vi "LSMcontroller_v66_improvedwfhandling.vi"() -> ()   [LabVIEW 2015] (continued)
                                tunnel: w3418 -> [_ w3423]
                                frame False {
                                }
                                frame True {
                                n926 = Quotient & Remainder(x=w3423, y=u32 2 ("min phot")) -> (floor(x/y)=w3422:u32)  [unwired: 1 out]
                                n927 = Max & Min(x=w3422, y=u32 5) -> (max(x,y)=w3421:u32)  [unwired: 1 out]
                                n928 = local write "min phot"(w3421) -> ()
                                }
                                }
                                n929 = To Double Precision Float(number=w3408) -> (double precision float=w3409:dbl)
                                n930 = local write "img_CH1"(w3410) -> ()
                                n931 = property on="img_CH1" class="IntGraph (strict)"("ZScale.Maximum"=w3409) -> ()  [unwired: 2 in, 2 out]
                                }
                                }
                                }
                                frame #4 {
                                w3427 = u16 1 items=["Stream to disk", "Post process", "real time process"] ("Ring")
                                n932 = local read "T3R Data processing"() -> (w3426:u16)
                                n933 = Equal?(x=w3426, y=w3427) -> (x = y?=w3425:bool)
                                n934 = case shown="False" w3425 {
                                frame False {
                                # "intensity"
                                n935 = local read "Current Average"() -> (w3432:sgl)
                                n936 = local read "image2list"() -> (w3428:u16)
                                n937 = local read "image1list"() -> (w3429:u16)
                                n938 = call "dattoimage.vi"("image2list"=w3428, "Current Average"=w3432, "image1list"=w3429) -> ("image 1 array out"=w3431:sgl[][])  [unwired: 1 out]
                                n939 = Transpose 2D Array(2D array=w3431) -> (transposed array=w3430:sgl[][])
                                n940 = local write "img_CH2"(w3430) -> ()
                                }
                                frame True {
                                }
                                }
                                }
                                }
                              }
                              frame Enabled {
                              }
                            }
                          }
                        }
                        n941 = local write "64bit disabled"(TRUE ("64bit disabled")) -> ()
                      }
                      frame #9 {
                        n942 = call "2pparameters.vi"("command"="get") -> ("params out"=w3435:T10)  [unwired: 1 in]
                        n943 = Unbundle By Name(w3435) -> ("auto OD"=w3434:bool)
                        n944 = case shown="True" w3434 {
                          frame False {
                          }
                          frame True {
                            n945 = call "configuration.vi"("command"="get") -> ("config out"=w3438:T11)  [unwired: 2 in, 1 out]
                            n946 = call "2pparameters.vi"("command"="get") -> ("params out"=w3441:T10)  [unwired: 1 in]
                            n947 = Unbundle By Name(w3438) -> ("image OD"=w3436:u16)
                            n948 = Unbundle By Name(w3441) -> ("ODfilt"=w3437:u16)
                            n949 = call "filterwheelcontrol_nothorlabslib.vi"("Current OD filt"=w3436, "New ODfilt"=w3437) -> ()  [unwired: 1 in]
                          }
                        }
                        n950 = call "reset AO_DO_v3.vi"() -> ()  [unwired: 12 in]
                      }
                      frame #10 {
                        n951 = stacked-sequence {
                          tunnel: w3455 -> [w3458 _ _ _ _ _]
                          tunnel: w3454 -> [w3457 _ _ _ _ _]
                          tunnel: w3453 -> [w3456 _ _ _ _ _]
                          tunnel: w3452 -> [_ w3507 _ _ _ _]
                          tunnel: w3451 -> [_ w3506 w3561 w3658 _ _]
                          tunnel: w3450 -> [_ w3505 w3560 w3657 _ _]
                          tunnel: w3449 -> [_ _ w3559 _ _ _]
                          tunnel: w3448 -> [_ _ w3558 _ _ _]
                          tunnel: w3447 -> [_ _ _ w3656 _ _]
                          tunnel: w3446 -> [_ _ _ w3655 _ _]
                          tunnel: w3445 -> [_ _ w3556 _ _ _]
                          tunnel: w3444 -> [_ _ w3555 _ _ _]
                          tunnel: w3443 -> [_ _ _ w3653 _ _]
                          tunnel: w3442 -> [_ _ _ w3652 _ _]
                          frame #0 {
                            n952 = case shown="False" w3458 {
                              tunnel: w3457 -> [_ w3480]
                              tunnel: w3456 -> [_ w3479]
                              frame True {
                                n953 = stacked-sequence {
                                seq-local: [w3459 _ _] -> [_ w3471 w3476]
                                frame #0 {
                                n954 = call "configuration.vi"("command"="get") -> ("config out"=w3465:T11)  [unwired: 2 in, 1 out]
                                n955 = Unbundle By Name(w3465) -> ("Voltage to Xgalvo"=w3462:i32)
                                n956 = call "2pparameters.vi"("command"="get") -> ("params out"=w3463:T10)  [unwired: 1 in]
                                n957 = in-place {
                                in-place-border: w3462 -> [w3470]
                                in-place-border: [w3467] -> w3459
                                n958 = in-place-cluster #9(w3463) -> ("aAO"=w3469:u32[])
                                n959 = call "remove channel from active arrayv2.vi"("line array in"=w3469, "line to remove"=w3470) -> ("line array out"=w3468:u32[], "index"=w3467:i32)  [unwired: 1 out]
                                n960 = in-place-cluster #9("aAO"=w3468) -> (w3460:T10)
                                }
                                n961 = call "2pparameters.vi"("Params in"=w3460, "command"="set") -> ()  [unwired: 1 out]
                                }
                                frame #1 {
                                n962 = call "waveformparamsv2.vi"("command"="rem AO", "index"=w3471) -> ()  [unwired: 3 in, 3 out]
                                }
                                frame #2 {
                                n963 = call "waveformsAObuffer.vi"("command"="get") -> ("AO wf out"=w3477:waveform(dbl)[])  [unwired: 1 in]
                                n964 = Delete From Array(array=w3477, length=1, index=w3476) -> (array with subset deleted=w3473:waveform(dbl)[])  [unwired: 1 out]
                                n965 = call "waveformsAObuffer.vi"("AO wf in"=w3473, "command"="set") -> ()  [unwired: 1 out]
                                }
                                }
                              }
                              frame False {
                                n966 = stacked-sequence {
                                seq-local: [w3481 _ _] -> [_ w3489 w3500]
                                tunnel: w3480 -> [_ w3488 _]
                                tunnel: w3479 -> [_ _ w3499]
                                frame #0 {
                                n967 = call "configuration.vi"("command"="get") -> ("config out"=w3486:T11)  [unwired: 2 in, 1 out]
                                n968 = Unbundle By Name(w3486) -> ("Voltage to Xgalvo"=w3482:i32)
                                n969 = call "2pparameters.vi"("command"="get") -> ("params out"=w3485:T10)  [unwired: 1 in]
                                n970 = Unbundle By Name(w3485) -> ("aAO"=w3483:u32[])
                                n971 = Search 1D Array(1D array=w3483, element=w3482) -> (index of element=w3481:i32)  [unwired: 1 in]
                                }
                                frame #1 {
                                n972 = call "waveformparamsv2.vi"("command"="get") -> ("Params out"=w3492:T14)  [unwired: 4 in, 2 out]
                                n973 = in-place {
                                in-place-border: w3489 -> [w3496]
                                in-place-border: w3488 -> [w3495]
                                n974 = in-place-cluster #10(w3492) -> ("AO parameters"=w3497:T15)
                                n975 = in-place {
                                in-place-border: w3495 -> [w3498]
                                n976 = in-place-array #11(w3497, w3496) -> ()  [unwired: 1 out]
                                n977 = in-place-array #11(w3498) -> (w3494:T15)  [unwired: 1 out]
                                }
                                n978 = in-place-cluster #10("AO parameters"=w3494) -> (w3490:T14)
                                }
                                n979 = call "waveformparamsv2.vi"("command"="set", "Params in"=w3490) -> ()  [unwired: 3 in, 3 out]
                                }
                                frame #2 {
                                n980 = call "waveformsAObuffer.vi"("command"="get") -> ("AO wf out"=w3503:waveform(dbl)[])  [unwired: 1 in]
                                n981 = Replace Array Subset(array=w3503, new element=w3499, index=w3500) -> (w3501:waveform(dbl)[])
                                n982 = call "waveformsAObuffer.vi"("AO wf in"=w3501, "command"="set") -> ()  [unwired: 1 out]
                                }
                                }
                              }
                            }
                          }
                          frame #1 {
                            n983 = case shown="True" w3507 {
                              tunnel: w3506 -> [_ w3529]
                              tunnel: w3505 -> [_ w3528]
                              frame True {
                                n984 = stacked-sequence {
                                seq-local: [w3508 _ _] -> [_ w3520 w3525]
                                frame #0 {
                                n985 = call "configuration.vi"("command"="get") -> ("config out"=w3514:T11)  [unwired: 2 in, 1 out]
                                n986 = Unbundle By Name(w3514) -> ("Voltage to Ygalvo"=w3511:i32)
                                n987 = call "2pparameters.vi"("command"="get") -> ("params out"=w3512:T10)  [unwired: 1 in]
                                n988 = in-place {
                                in-place-border: w3511 -> [w3519]
                                in-place-border: [w3516] -> w3508
                                n989 = in-place-cluster #12(w3512) -> ("aAO"=w3518:u32[])
                                n990 = call "remove channel from active arrayv2.vi"("line array in"=w3518, "line to remove"=w3519) -> ("line array out"=w3517:u32[], "index"=w3516:i32)  [unwired: 1 out]
                                n991 = in-place-cluster #12("aAO"=w3517) -> (w3509:T10)
                                }
                                n992 = call "2pparameters.vi"("Params in"=w3509, "command"="set") -> ()  [unwired: 1 out]
                                }
                                frame #1 {
                                n993 = call "waveformparamsv2.vi"("command"="rem AO", "index"=w3520) -> ()  [unwired: 3 in, 3 out]
                                }
                                frame #2 {
                                n994 = call "waveformsAObuffer.vi"("command"="get") -> ("AO wf out"=w3526:waveform(dbl)[])  [unwired: 1 in]
                                n995 = Delete From Array(array=w3526, length=1, index=w3525) -> (array with subset deleted=w3522:waveform(dbl)[])  [unwired: 1 out]
                                n996 = call "waveformsAObuffer.vi"("AO wf in"=w3522, "command"="set") -> ()  [unwired: 1 out]
                                }
                                }
                              }
                              frame False {
                                n997 = stacked-sequence {
                                seq-local: [w3530 _ _] -> [_ w3538 w3549]
                                tunnel: w3529 -> [_ w3537 _]
                                tunnel: w3528 -> [_ _ w3548]
                                frame #0 {
                                n998 = call "configuration.vi"("command"="get") -> ("config out"=w3535:T11)  [unwired: 2 in, 1 out]
                                n999 = Unbundle By Name(w3535) -> ("Voltage to Ygalvo"=w3531:i32)
                                n1000 = call "2pparameters.vi"("command"="get") -> ("params out"=w3534:T10)  [unwired: 1 in]
                                n1001 = Unbundle By Name(w3534) -> ("aAO"=w3532:u32[])
                                n1002 = Search 1D Array(1D array=w3532, element=w3531) -> (index of element=w3530:i32)  [unwired: 1 in]
                                }
                                frame #1 {
                                n1003 = call "waveformparamsv2.vi"("command"="get") -> ("Params out"=w3541:T14)  [unwired: 4 in, 2 out]
                                n1004 = in-place {
                                in-place-border: w3538 -> [w3545]
                                in-place-border: w3537 -> [w3544]
                                n1005 = in-place-cluster #13(w3541) -> ("AO parameters"=w3546:T15)
                                n1006 = in-place {
                                in-place-border: w3544 -> [w3547]
                                n1007 = in-place-array #14(w3546, w3545) -> ()  [unwired: 1 out]
                                n1008 = in-place-array #14(w3547) -> (w3543:T15)  [unwired: 1 out]
                                }
                                n1009 = in-place-cluster #13("AO parameters"=w3543) -> (w3539:T14)
                                }
                                n1010 = call "waveformparamsv2.vi"("command"="set", "Params in"=w3539) -> ()  [unwired: 3 in, 3 out]
                                }
                                frame #2 {
                                n1011 = call "waveformsAObuffer.vi"("command"="get") -> ("AO wf out"=w3552:waveform(dbl)[])  [unwired: 1 in]
                                n1012 = Replace Array Subset(array=w3552, new element=w3548, index=w3549) -> (w3550:waveform(dbl)[])
                                n1013 = call "waveformsAObuffer.vi"("AO wf in"=w3550, "command"="set") -> ()  [unwired: 1 out]
                                }
                                }
                              }
                            }
                          }
                          frame #2 {
                            n1014 = Build Array(w3556, w3555) -> (w3554:bool[])
                            n1015 = Boolean Array To Number(Boolean array=w3554) -> (number=w3557:u32)
                            n1016 = case shown="0" w3557 {
                              tunnel: w3561 -> [_ _ w3604]
                              tunnel: w3560 -> [_ _ w3603]
                              tunnel: w3559 -> [_ w3583 w3601]
                              tunnel: w3558 -> [_ w3582 w3602]
                              frame 1, Default {
                                n1017 = stacked-sequence {
                                seq-local: [w3562 _ _] -> [_ w3574 w3579]
                                frame #0 {
                                n1018 = call "configuration.vi"("command"="get") -> ("config out"=w3568:T11)  [unwired: 2 in, 1 out]
                                n1019 = Unbundle By Name(w3568) -> ("2P shutter"=w3565:i32)
                                n1020 = call "2pparameters.vi"("command"="get") -> ("params out"=w3566:T10)  [unwired: 1 in]
                                n1021 = in-place {
                                in-place-border: w3565 -> [w3573]
                                in-place-border: [w3570] -> w3562
                                n1022 = in-place-cluster #15(w3566) -> ("aDO"=w3572:u32[])
                                n1023 = call "remove channel from active arrayv2.vi"("line array in"=w3572, "line to remove"=w3573) -> ("line array out"=w3571:u32[], "index"=w3570:i32)  [unwired: 1 out]
                                n1024 = in-place-cluster #15("aDO"=w3571) -> (w3563:T10)
                                }
                                n1025 = call "2pparameters.vi"("Params in"=w3563, "command"="set") -> ()  [unwired: 1 out]
                                }
                                frame #1 {
                                n1026 = call "waveformparamsv2.vi"("command"="rem DO", "index"=w3574) -> ()  [unwired: 3 in, 3 out]
                                }
                                frame #2 {
                                n1027 = call "waveformsDObuffer.vi"("command"="get") -> ("DO wf out"=w3580:digitalwaveform[])  [unwired: 1 in]
                                n1028 = Delete From Array(array=w3580, length=1, index=w3579) -> (array with subset deleted=w3576:digitalwaveform[])  [unwired: 1 out]
                                n1029 = call "waveformsDObuffer.vi"("DO wf in"=w3576, "command"="set") -> ()  [unwired: 1 out]
                                }
                                }
                              }
                              frame 2 {
                                n1030 = stacked-sequence {
                                tunnel: w3583 -> [_ w3594 _]
                                tunnel: w3582 -> [_ _ w3598]
                                frame #0 {
                                n1031 = call "configuration.vi"("command"="get") -> ("config out"=w3585:T11)  [unwired: 2 in, 1 out]
                                n1032 = call "2pparameters.vi"("command"="get") -> ("params out"=w3589:T10)  [unwired: 1 in]
                                n1033 = Unbundle By Name(w3585) -> ("2P shutter"=w3584:i32)
                                n1034 = in-place {
                                in-place-border: w3584 -> [w3593]
                                n1035 = in-place-cluster #16(w3589) -> ("aDO"=w3592:u32[])
                                n1036 = call "add channel to active arrayv2.vi"("line array in"=w3592, "line to add"=w3593) -> ("line array out"=w3591:u32[])  [unwired: 2 out]
                                n1037 = in-place-cluster #16("aDO"=w3591) -> (w3587:T10)
                                }
                                n1038 = call "2pparameters.vi"("Params in"=w3587, "command"="set") -> ()  [unwired: 1 out]
                                }
                                frame #1 {
                                n1039 = call "waveformparamsv2.vi"("command"="add DO", "add DO"=w3594) -> ()  [unwired: 3 in, 3 out]
                                }
                                frame #2 {
                                n1040 = call "waveformsDObuffer.vi"("command"="get") -> ("DO wf out"=w3599:digitalwaveform[])  [unwired: 1 in]
                                n1041 = Build Array (concatenate)(w3599, w3598) -> (w3597:digitalwaveform[])
                                n1042 = call "waveformsDObuffer.vi"("DO wf in"=w3597, "command"="set") -> ()  [unwired: 1 out]
                                }
                                }
                              }
                              frame 0 {
                                n1043 = stacked-sequence {
                                seq-local: [w3605 _ _] -> [_ w3613 w3635]
                                tunnel: w3604 -> [_ _ _]
                                tunnel: w3603 -> [_ _ _]
                                tunnel: w3602 -> [_ _ w3634]
                                tunnel: w3601 -> [_ w3612 _]
                                frame #0 {
                                n1044 = call "configuration.vi"("command"="get") -> ("config out"=w3610:T11)  [unwired: 2 in, 1 out]
                                n1045 = call "2pparameters.vi"("command"="get") -> ("params out"=w3609:T10)  [unwired: 1 in]
                                n1046 = Unbundle By Name(w3610) -> ("2P shutter"=w3606:i32)
                                n1047 = Unbundle By Name(w3609) -> ("aDO"=w3607:u32[])
                                n1048 = Search 1D Array(1D array=w3607, element=w3606) -> (index of element=w3605:i32)  [unwired: 1 in]
                                }
                                frame #1 {
                                n1049 = call "2pparameters.vi"("command"="get") -> ("params out"=w3616:T10)  [unwired: 1 in]
                                n1050 = Unbundle By Name(w3616) -> ("wavdet"=w3614:bool, "autoshutter"=w3615:bool)
                                n1051 = case shown="True" w3615 {
                                tunnel: w3613 -> [_ w3620]
                                tunnel: w3614 -> [_ w3619]
                                tunnel: w3612 -> [_ w3618]
                                frame False {
                                }
                                frame True {
                                n1052 = case shown="False" w3619 {
                                tunnel: w3620 -> [w3624 _]
                                tunnel: w3618 -> [w3622 _]
                                frame False {
                                n1053 = Index Array(array=w3622, index=0) -> (element=w3621:T18)
                                n1054 = call "waveformparamsv2.vi"("command"="get") -> ("Params out"=w3627:T14)  [unwired: 4 in, 2 out]
                                n1055 = in-place {
                                in-place-border: w3624 -> [w3631]
                                in-place-border: w3621 -> [w3629]
                                n1056 = in-place-cluster #17(w3627) -> ("DO parameters"=w3632:T17)
                                n1057 = in-place {
                                in-place-border: w3629 -> [w3633]
                                n1058 = in-place-array #18(w3632, w3631) -> ()  [unwired: 1 out]
                                n1059 = in-place-array #18(w3633) -> (w3630:T17)  [unwired: 1 out]
                                }
                                n1060 = in-place-cluster #17("DO parameters"=w3630) -> (w3625:T14)
                                }
                                n1061 = call "waveformparamsv2.vi"("command"="set", "Params in"=w3625) -> ()  [unwired: 3 in, 3 out]
                                }
                                frame True {
                                }
                                }
                                }
                                }
                                }
                                frame #2 {
                                n1062 = call "2pparameters.vi"("command"="get") -> ("params out"=w3638:T10)  [unwired: 1 in]
                                n1063 = Unbundle By Name(w3638) -> ("wavdet"=w3636:bool, "autoshutter"=w3637:bool)
                                n1064 = case shown="True" w3637 {
                                tunnel: w3635 -> [_ w3642]
                                tunnel: w3636 -> [_ w3641]
                                tunnel: w3634 -> [_ w3640]
                                frame False {
                                }
                                frame True {
                                n1065 = case shown="False" w3641 {
                                tunnel: w3642 -> [w3646 _]
                                tunnel: w3640 -> [w3645 _]
                                frame False {
                                n1066 = Index Array(array=w3645, index=0) -> (element=w3643:digitalwaveform)
                                n1067 = call "waveformsDObuffer.vi"("command"="get") -> ("DO wf out"=w3648:digitalwaveform[])  [unwired: 1 in]
                                n1068 = Replace Array Subset(array=w3648, new element=w3643, index=w3646) -> (w3650:digitalwaveform[])
                                n1069 = call "waveformsDObuffer.vi"("DO wf in"=w3650, "command"="set") -> ()  [unwired: 1 out]
                                }
                                frame True {
                                }
                                }
                                }
                                }
                                }
                                }
                              }
                            }
                          }
                          frame #3 {
                            n1070 = Build Array(w3653, w3652) -> (w3654:bool[])
                            n1071 = Boolean Array To Number(Boolean array=w3654) -> (number=w3651:u32)
                            n1072 = case shown="0" w3651 {
                              tunnel: w3658 -> [_ _ w3701]
                              tunnel: w3657 -> [_ _ w3700]
                              tunnel: w3656 -> [_ w3680 w3698]
                              tunnel: w3655 -> [_ w3679 w3699]
                              frame 1, Default {
                                n1073 = stacked-sequence {
                                seq-local: [w3659 _ _] -> [_ w3671 w3676]
                                frame #0 {
                                n1074 = call "configuration.vi"("command"="get") -> ("config out"=w3665:T11)  [unwired: 2 in, 1 out]
                                n1075 = Unbundle By Name(w3665) -> ("LT timestamp"=w3662:u32)
                                n1076 = call "2pparameters.vi"("command"="get") -> ("params out"=w3663:T10)  [unwired: 1 in]
                                n1077 = in-place {
                                in-place-border: w3662 -> [w3670]
                                in-place-border: [w3667] -> w3659
                                n1078 = in-place-cluster #19(w3663) -> ("aDO"=w3669:u32[])
                                n1079 = call "remove channel from active arrayv2.vi"("line array in"=w3669, "line to remove"=w3670) -> ("line array out"=w3668:u32[], "index"=w3667:i32)  [unwired: 1 out]
                                n1080 = in-place-cluster #19("aDO"=w3668) -> (w3660:T10)
                                }
                                n1081 = call "2pparameters.vi"("Params in"=w3660, "command"="set") -> ()  [unwired: 1 out]
                                }
                                frame #1 {
                                n1082 = call "waveformparamsv2.vi"("command"="rem DO", "index"=w3671) -> ()  [unwired: 3 in, 3 out]
                                }
                                frame #2 {
                                n1083 = call "waveformsDObuffer.vi"("command"="get") -> ("DO wf out"=w3677:digitalwaveform[])  [unwired: 1 in]
                                n1084 = Delete From Array(array=w3677, length=1, index=w3676) -> (array with subset deleted=w3673:digitalwaveform[])  [unwired: 1 out]
                                n1085 = call "waveformsDObuffer.vi"("DO wf in"=w3673, "command"="set") -> ()  [unwired: 1 out]
                                }
                                }
                              }
                              frame 2 {
                                n1086 = stacked-sequence {
                                tunnel: w3680 -> [_ _ w3693]
                                tunnel: w3679 -> [_ w3691 _]
                                frame #0 {
                                n1087 = call "configuration.vi"("command"="get") -> ("config out"=w3682:T11)  [unwired: 2 in, 1 out]
                                n1088 = Unbundle By Name(w3682) -> ("LT timestamp"=w3681:u32)
                                n1089 = call "2pparameters.vi"("command"="get") -> ("params out"=w3686:T10)  [unwired: 1 in]
                                n1090 = in-place {
                                in-place-border: w3681 -> [w3690]
                                n1091 = in-place-cluster #20(w3686) -> ("aDO"=w3689:u32[])
                                n1092 = call "add channel to active arrayv2.vi"("line array in"=w3689, "line to add"=w3690) -> ("line array out"=w3688:u32[])  [unwired: 2 out]
                                n1093 = in-place-cluster #20("aDO"=w3688) -> (w3684:T10)
                                }
                                n1094 = call "2pparameters.vi"("Params in"=w3684, "command"="set") -> ()  [unwired: 1 out]
                                }
                                frame #1 {
                                n1095 = call "waveformparamsv2.vi"("command"="add DO", "add DO"=w3691) -> ()  [unwired: 3 in, 3 out]
                                }
                                frame #2 {
                                n1096 = call "waveformsDObuffer.vi"("command"="get") -> ("DO wf out"=w3696:digitalwaveform[])  [unwired: 1 in]
                                n1097 = Build Array (concatenate)(w3696, w3693) -> (w3695:digitalwaveform[])
                                n1098 = call "waveformsDObuffer.vi"("DO wf in"=w3695, "command"="set") -> ()  [unwired: 1 out]
                                }
                                }
                              }
                              frame 0 {
                                n1099 = stacked-sequence {
                                seq-local: [w3702 _ _] -> [_ w3712 w3729]
                                tunnel: w3701 -> [_ _ _]
                                tunnel: w3700 -> [_ _ _]
                                tunnel: w3699 -> [_ w3709 _]
                                tunnel: w3698 -> [_ _ w3728]
                                frame #0 {
                                n1100 = call "configuration.vi"("command"="get") -> ("config out"=w3707:T11)  [unwired: 2 in, 1 out]
                                n1101 = Unbundle By Name(w3707) -> ("LT timestamp"=w3703:u32)
                                n1102 = call "2pparameters.vi"("command"="get") -> ("params out"=w3706:T10)  [unwired: 1 in]
                                n1103 = Unbundle By Name(w3706) -> ("aDO"=w3704:u32[])
                                n1104 = Search 1D Array(1D array=w3704, element=w3703) -> (index of element=w3702:i32)  [unwired: 1 in]
                                }
                                frame #1 {
                                n1105 = local read "Measurement"() -> (w3711:T4)
                                n1106 = To Unsigned Long Integer(number=w3711) -> (unsigned 32bit integer=w3710:u32)
                                n1107 = case shown="5..7" w3710 {
                                tunnel: w3712 -> [_ w3716]
                                tunnel: w3709 -> [_ w3713]
                                frame 0..4, Default {
                                }
                                frame 5..7 {
                                n1108 = Index Array(array=w3713, index=0) -> (element=w3714:T18)
                                n1109 = call "waveformparamsv2.vi"("command"="get") -> ("Params out"=w3719:T14)  [unwired: 4 in, 2 out]
                                n1110 = in-place {
                                in-place-border: w3716 -> [w3723]
                                in-place-border: w3714 -> [w3721]
                                n1111 = in-place-cluster #21(w3719) -> ("DO parameters"=w3724:T17)
                                n1112 = in-place {
                                in-place-border: w3721 -> [w3725]
                                n1113 = in-place-array #22(w3724, w3723) -> ()  [unwired: 1 out]
                                n1114 = in-place-array #22(w3725) -> (w3722:T17)  [unwired: 1 out]
                                }
                                n1115 = in-place-cluster #21("DO parameters"=w3722) -> (w3717:T14)
                                }
                                n1116 = call "waveformparamsv2.vi"("command"="set", "Params in"=w3717) -> ()  [unwired: 3 in, 3 out]
                                }
                                }
                                }
                                frame #2 {
                                n1117 = local read "Measurement"() -> (w3727:T4)
                                n1118 = To Unsigned Long Integer(number=w3727) -> (unsigned 32bit integer=w3726:u32)
                                n1119 = case shown="5..7" w3726 {
                                tunnel: w3729 -> [_ w3733]
                                tunnel: w3728 -> [_ w3731]
                                frame 0..4, Default {
                                }
                                frame 5..7 {
                                n1120 = Index Array(array=w3731, index=0) -> (element=w3730:digitalwaveform)
                                n1121 = call "waveformsDObuffer.vi"("command"="get") -> ("DO wf out"=w3735:digitalwaveform[])  [unwired: 1 in]
                                n1122 = Replace Array Subset(array=w3735, new element=w3730, index=w3733) -> (w3737:digitalwaveform[])
                                n1123 = call "waveformsDObuffer.vi"("DO wf in"=w3737, "command"="set") -> ()  [unwired: 1 out]
                                }
                                }
                                }
                                }
                              }
                            }
                          }
                          frame #4 {
                            n1124 = call "Used AO lines.vi"() -> ("used AO names"=w3740:string[], "used AO lines"=w3738:tag[])  [unwired: 2 in]
                            n1125 = control-ref of="Analog Lines Plot"() -> (w3739:refnum<vi>)
                            n1126 = control-ref of="Digital Lines Plot"() -> (w3741:refnum<vi>)
                            n1127 = call "Used DO lines.vi"() -> ("used DO names"=w3742:string[], "used DO lines"=w3743:tag[])  [unwired: 2 in]
                            n1128 = local write "Analog Used Lines"(w3738) -> ()
                            n1129 = local write "Analog Used Names"(w3740) -> ()
                            n1130 = local write "Digital Used Lines"(w3743) -> ()
                            n1131 = local write "Digital Used Names"(w3742) -> ()
                            n1132 = call "prepDOWaveplot.vi"("DigitalGraph in"=w3741, "used DO names"=w3742) -> ()  [unwired: 1 in]
                            n1133 = call "prepAOWaveplot.vi"("WaveformGraph in"=w3739, "Analog Used Names"=w3740) -> ()  [unwired: 1 in]
                          }
                          frame #5 {
                            n1134 = local read "Meastab"() -> (w3758:enum32{"X-Y Image", "Linescan", "Timetrace"})
                            n1135 = property on="refwf" class="Ring (strict)"() -> ("RingText.Text"=w3755:string)  [unwired: 2 in, 2 out]
                            n1136 = case shown="\"Timetrace\"" w3758 {
                              tunnel: [w3760 w3761] -> w3759
                              frame "X-Y Image", Default {
                                n1137 = local read "Sampling rate"() -> (w3760:dbl)
                              }
                              frame "Timetrace" {
                                n1138 = local read "srateAODOtt"() -> (w3761:dbl)
                              }
                            }
                            n1139 = call "waveformsAObuffer.vi"("command"="get") -> ("AO wf out"=w3746:waveform(dbl)[])  [unwired: 1 in]
                            n1140 = local read "wavdet"() -> (w3756:bool)
                            n1141 = call "waveformsDObuffer.vi"("command"="get") -> ("DO wf out"=w3750:digitalwaveform[])  [unwired: 1 in]
                            n1142 = call "correctwaveformsizetemp.vi"("new sampling frequency (Hz)"=w3759, "start"=FALSE, "reference waveforms to"=w3755, "Analog waveforms in"=w3746, "stop"=TRUE, "Digital waveforms in"=w3750) -> ("analog wf out"=w3752:waveform(dbl)[], "Digital wf out"=w3754:digitalwaveform[], "measpoints"=w3757:i32)
                            n1143 = local write "Analog Lines Plot"(w3752) -> ()
                            n1144 = call "GetNumCamFramesv2.vi"("Digital Waveform Graph"=w3754) -> ("Numeric"=w3753:i32)  [unwired: 10 in]
                            n1145 = local write "Digital Lines Plot"(w3754) -> ()
                            n1146 = call "waveformsDObuffer.vi"("DO wf in"=w3754, "command"="set") -> ()  [unwired: 1 out]
                            n1147 = call "waveformsAObuffer.vi"("AO wf in"=w3752, "command"="set") -> ()  [unwired: 1 out]
                            n1148 = local write "Total Camera Frames"(w3753) -> ()
                            n1149 = case shown="True" w3756 {
                              tunnel: w3757 -> [_ w3762]
                              frame False {
                              }
                              frame True {
                                n1150 = local write "# of frames"(w3762) -> ()
                              }
                            }
                          }
                        }
                        n1151 = call "stoperaseCI.vi"() -> ()  [unwired: 12 in]
                        n1152 = call "stoperaseDO_img.vi"() -> ()  [unwired: 12 in]
                        n1153 = call "stoperaseAO_img.vi"() -> ()  [unwired: 12 in]
                        n1154 = call "stoperaseAI_img.vi"() -> ()  [unwired: 12 in]
                      }
                      frame #11 {
                        w3770 = FALSE ("Value (Signaling)")
                        n1155 = local read "save\ndata"() -> (w3763:bool)
                        n1156 = local read "save\ndata"() -> (w3764:bool)
                        n1157 = property on="Stop" class="Bool (strict)"("Visible"=FALSE, "DisabledEnum"=T7."Disabled" ("Disabled")) -> ()  [unwired: 2 in, 2 out]
                        n1158 = case shown="True" w3763 {
                          frame False {
                          }
                          frame True {
                            n1159 = call "closetiffs.vi"() -> ()  [unwired: 12 in]
                          }
                        }
                        n1160 = case shown="True" w3764 {
                          tunnel: w3765 -> [_ w3771]
                          frame False {
                          }
                          frame True {
                            n1161 = local read "filename prefix"() -> (w3773:string)
                            n1162 = local read "data dir"() -> (w3772:path)
                            n1163 = call "savetimestamps.vi"("timestamp"=w3771, "filename prefix in"=w3773, "data dir in"=w3772) -> ()  [unwired: 1 in]
                            n1164 = call "saveparams.vi"("filename prefix in"=w3773, "data dir in"=w3772) -> ()  [unwired: 2 in]
                          }
                        }
                        n1165 = property on="Start" class="Bool (strict)"("Visible"=TRUE, "DisabledEnum"=T7."Enabled" ("Disabled")) -> ()  [unwired: 2 in, 2 out]
                        n1166 = property on="Start" class="Bool (strict)"("Val(Sgnl)"=w3770) -> ()  [unwired: 2 in, 2 out]
                        n1167 = property on="Stop" class="Bool (strict)"("Val(Sgnl)"=w3770) -> ()  [unwired: 2 in, 2 out]
                      }
                      frame #12 {
                        w3777 = T21 2 items=["no dialog", "OK message", "continue or stop message", "OK message + warnings", "continue/stop + warnings"] ("type of dialog (OK msg:1)")
                        n1168 = call "displayerrors.vi"() -> ("error IO"=w3776:errorcluster)
                        n1169 = call <vilib>:"General Error Handler.vi"("type of dialog (OK msg:1)"=w3777, "error in (no error)"=w3776) -> ("error out"=w3775:errorcluster)  [unwired: 9 in, 4 out]
                        n1170 = call <vilib>:"Clear Errors.vi"("error in (no error)"=w3775) -> ("error out"=w3774:errorcluster)  [unwired: 5 in, 1 out]
                        n1171 = call "seterrors.vi"("error IO"=w3774) -> ()
                      }
                    }
                  }
                  frame "X-Y-Z-t movie" {
                    n1172 = call "2pparameters.vi"("command"="get") -> ("params out"=w3780:T10)  [unwired: 1 in]
                    n1173 = Bundle By Name(cluster=w3780, "type"="X-Y-Z-t movie") -> (w3778:T10)
                    n1174 = call "2pparameters.vi"("Params in"=w3778, "command"="set") -> ()  [unwired: 1 out]
                  }
                  frame "linescan" {
                    n1175 = call "2pparameters.vi"("command"="get") -> ("params out"=w3785:T10)  [unwired: 1 in]
                    n1176 = Bundle By Name(cluster=w3785, "type"="linescan") -> (w3787:T10)
                    n1177 = call "2pparameters.vi"("Params in"=w3787, "command"="set") -> ()  [unwired: 1 out]
                  }
                  frame "Timetrace", "Lifetime (contour)" {
                    n1178 = local read "ttt"() -> (w3788:T3)
                    n1179 = case shown="\"Point\", \"Resonant Ellipse\", \"freeform contour\", \"Fill Ellipse\", Default" w3788 {
                      selector: w3788 -> [_ w3789]
                      frame "Line" {
                      }
                      frame "Point", "Resonant Ellipse", "freeform contour", "Fill Ellipse", Default {
                        n1180 = stacked-sequence {
                          seq-local: [w3805 _ _ _ _ _ _ _ _ _ _] -> [_ _ w4678 _ _ w4691 w4758 _ _ w5118 _]
                          seq-local: [w3804 _ _ _ _ _ _ _ _ _ _] -> [_ _ _ _ _ _ _ _ w4805 _ _]
                          seq-local: [w3803 _ _ _ _ _ _ _ _ _ _] -> [_ _ _ _ _ _ _ _ w4804 _ _]
                          seq-local: [w3802 _ _ _ _ _ _ _ _ _ _] -> [_ _ _ _ _ _ _ _ w4807 _ _]
                          seq-local: [w3801 _ _ _ _ _ _ _ _ _ _] -> [_ _ _ _ _ _ _ _ w4803 _ _]
                          seq-local: [w3800 _ _ _ _ _ _ _ _ _ _] -> [_ _ _ _ _ _ _ _ w4802 _ _]
                          seq-local: [w3799 _ _ _ _ _ _ _ _ _ _] -> [_ _ _ _ _ _ _ _ w4806 _ _]
                          seq-local: [w3798 _ _ _ _ _ _ _ _ _ _] -> [_ _ _ _ _ _ _ _ w4801 _ _]
                          seq-local: [w3797 _ _ _ _ _ _ _ _ _ _] -> [_ _ _ _ _ _ _ _ w4800 _ _]
                          seq-local: [w3796 _ _ _ _ _ _ _ _ _ _] -> [_ _ _ _ _ _ _ _ w4795 _ _]
                          seq-local: [w3795 _ _ _ _ _ _ _ _ _ _] -> [_ _ _ _ _ _ _ _ w4794 _ _]
                          seq-local: [w3794 _ _ _ _ _ _ _ _ _ _] -> [_ _ _ _ _ _ _ _ w4799 _ _]
                          seq-local: [w3793 _ _ _ _ _ _ _ _ _ _] -> [_ _ _ _ _ _ _ _ w4798 _ _]
                          seq-local: [w3792 _ _ _ _ _ _ _ _ _ _] -> [_ _ _ _ _ _ _ _ w4797 _ _]
                          seq-local: [w3791 _ _ _ _ _ _ _ _ _ _] -> [_ _ _ _ _ _ _ _ w4796 _ _]
                          tunnel: w3789 -> [w3790 _ _ _ _ _ _ _ _ _ _]
                          frame #0 {
                            n1181 = local read "save\ndata"() -> (w3806:bool)
                            n1182 = Get Date/Time In Seconds() -> (seconds since 1Jan1904=w3807:timestamp)
                            n1183 = case shown="False" w3806 {
                              tunnel: w3807 -> [w3808 w3810]
                              tunnel: [w3808 w3809] -> w3805
                              frame False {
                              }
                              frame True {
                                n1184 = call "createdatafolder.vi"("timestamp in"=w3810) -> ("current data path"=w3811:path, "timestamp out"=w3809:timestamp)
                                n1185 = local write "data dir"(w3811) -> ()
                              }
                            }
                            n1186 = stacked-sequence {
                              tunnel: w3805 -> [w3817 _ _ _ _ _ _ _ _]
                              tunnel: [_ _ _ _ _ _ w3983 _ _] -> w3804
                              tunnel: [_ _ _ _ _ _ w3982 _ _] -> w3803
                              tunnel: [_ _ _ _ _ _ w3981 _ _] -> w3802
                              tunnel: [_ _ _ _ _ _ w3980 _ _] -> w3801
                              tunnel: [_ _ _ _ _ _ w3979 _ _] -> w3800
                              tunnel: [_ _ _ _ _ _ w3978 _ _] -> w3799
                              tunnel: [_ _ _ _ _ _ w3977 _ _] -> w3798
                              tunnel: [_ _ _ _ _ _ w3976 _ _] -> w3797
                              tunnel: [_ _ _ _ _ _ w3975 _ _] -> w3796
                              tunnel: [_ _ _ _ _ _ w3974 _ _] -> w3795
                              tunnel: [_ _ _ _ _ _ w3973 _ _] -> w3794
                              tunnel: [_ _ _ _ _ _ w3972 _ _] -> w3793
                              tunnel: [_ _ _ _ _ _ w3971 _ _] -> w3792
                              tunnel: [_ _ _ _ _ _ w3970 _ _] -> w3791
                              tunnel: w3790 -> [_ _ w3855 _ w3914 _ _ _ _]
                              frame #0 {
                                n1187 = local write "graphtab"(T5."timetrace" ("graphtab")) -> ()
                                n1188 = local read "AI channels"() -> (w3821:i32[])
                                n1189 = local read "CI channels"() -> (w3822:i32[])
                                n1190 = property on="Stop" class="Bool (strict)"("Visible"=TRUE, "DisabledEnum"=T7."Enabled" ("Disabled")) -> ()  [unwired: 2 in, 2 out]
                                n1191 = property on="Start" class="Bool (strict)"("Visible"=FALSE, "DisabledEnum"=T7."Disabled and Grayed Out" ("Disabled")) -> ()  [unwired: 2 in, 2 out]
                                n1192 = Format Date/Time String(time format string (%c)="%Y%m%d", seconds (now)=w3817) -> (date/time string=w3816:string)  [unwired: 1 in]
                                n1193 = Format Date/Time String(time format string (%c)="%H%M%S", seconds (now)=w3817) -> (date/time string=w3815:string)  [unwired: 1 in]
                                n1194 = call "2pparameters.vi"("command"="get") -> ("params out"=w3824:T10)  [unwired: 1 in]
                                n1195 = Bundle By Name(cluster=w3824, "aAI"=w3821, "aCI"=w3822, "type"="Timetrace", "date"=w3816, "time"=w3815) -> (w3823:T10)
                                n1196 = call "X-array-databuffer.vi"("command"=enum16{"get", "set", "clear", "append"}."clear") -> ()  [unwired: 3 in, 2 out]
                                n1197 = call "Y-array-databuffer.vi"("command"=enum16{"get", "set", "clear", "append"}."clear") -> ()  [unwired: 3 in, 2 out]
                                n1198 = call "2pparameters.vi"("Params in"=w3823, "command"="set") -> ()  [unwired: 1 out]
                                n1199 = call "CH1-1D-temp.vi"("command"=enum16{"get", "set", "clear", "append"}."clear") -> ()  [unwired: 3 in, 2 out]
                                n1200 = call "CH2-1D-temp.vi"("command"=enum16{"get", "set", "clear", "append"}."clear") -> ()  [unwired: 3 in, 2 out]
                                n1201 = call "allAI-temp.vi"("command"=enum16{"get", "set", "clear", "append"}."clear") -> ()  [unwired: 3 in, 2 out]
                              }
                              frame #1 {
                                n1202 = call "configuration.vi"("command"="get") -> ("config out"=w3841:T11)  [unwired: 2 in, 1 out]
                                n1203 = Unbundle By Name(w3841) -> ("CI names"=w3842:string[], "AI names"=w3843:string[])
                                n1204 = call "2pparameters.vi"("command"="get") -> ("params out"=w3837:T10)  [unwired: 1 in]
                                n1205 = Unbundle By Name(w3837) -> ("aCI"=w3838:i32[], "aAI"=w3839:i32[])
                                n1206 = for {
                                tunnel: w3838 -> [w3853] mode=indexing
                                tunnel: w3842 -> [w3854]
                                tunnel: [w3852] -> w3844 mode=indexing
                                n1207 = Index Array(array=w3854, index=w3853) -> (element=w3852:string)
                                }
                                n1208 = for {
                                tunnel: w3839 -> [w3850] mode=indexing
                                tunnel: w3843 -> [w3851]
                                tunnel: [w3849] -> w3845 mode=indexing
                                n1209 = Index Array(array=w3851, index=w3850) -> (element=w3849:string)
                                }
                                n1210 = Build Array (concatenate)(w3844, w3845) -> (w3835:string[])
                                n1211 = for {
                                tunnel: w3835 -> [w3847] mode=indexing
                                tunnel: [w3846] -> w3834 mode=indexing
                                i -> [w3848]
                                n1212 = Bundle("String"=w3847, w3848) -> (w3846:cluster{"String":string, i32})  [unwired: 1 in]
                                }
                                n1213 = property on="graph1list" class="Ring (strict)"("StringsAndValues[]"=w3834) -> ()  [unwired: 2 in, 2 out]
                                n1214 = property on="graph2list" class="Ring (strict)"("StringsAndValues[]"=w3834) -> ()  [unwired: 2 in, 2 out]
                              }
                              frame #2 {
                                n1215 = call "2pparameters.vi"("command"="get") -> ("params out"=w3858:T10)  [unwired: 1 in]
                                n1216 = Unbundle By Name(w3858) -> ("auto OD"=w3856:bool, "autoshutter"=w3859:bool)
                                n1217 = case shown="True" w3856 {
                                tunnel: w3855 -> [_ w3860]
                                frame False {
                                }
                                frame True {
                                n1218 = case shown="\"Point\"" w3860 {
                                frame "Point" {
                                n1219 = call "configuration.vi"("command"="get") -> ("config out"=w3863:T11)  [unwired: 2 in, 1 out]
                                n1220 = Unbundle By Name(w3863) -> ("point OD"=w3864:u16)
                                n1221 = local read "ODfilt"() -> (w3861:u16)
                                n1222 = call "filterwheelcontrol_nothorlabslib.vi"("Current OD filt"=w3861, "New ODfilt"=w3864) -> ()  [unwired: 1 in]
                                }
                                frame "Resonant Ellipse", Default {
                                n1223 = call "configuration.vi"("command"="get") -> ("config out"=w3867:T11)  [unwired: 2 in, 1 out]
                                n1224 = Unbundle By Name(w3867) -> ("contour OD"=w3868:u16)
                                n1225 = local read "ODfilt"() -> (w3865:u16)
                                n1226 = call "filterwheelcontrol_nothorlabslib.vi"("Current OD filt"=w3865, "New ODfilt"=w3868) -> ()  [unwired: 1 in]
                                }
                                }
                                }
                                }
                                n1227 = case shown="True" w3859 {
                                frame False {
                                }
                                frame True {
                                n1228 = call "shuttercontrol.vi"("command"="close") -> ()  [unwired: 1 in, 1 out]
                                }
                                }
                              }
                              frame #3 {
                                n1229 = local read "Vy-min draw"() -> (w3877:dbl)
                                n1230 = local read "Vy-max draw"() -> (w3876:dbl)
                                n1231 = local read "Vx-min draw"() -> (w3879:dbl)
                                n1232 = local read "Vx-max draw"() -> (w3878:dbl)
                                n1233 = local read "xpixels ref"() -> (w3875:i32)
                                n1234 = local read "ypixels ref"() -> (w3874:i32)
                                n1235 = local read "ROI Type"() -> (w3873:u16)
                                n1236 = local read "srateAODOtt"() -> (w3896:dbl)
                                n1237 = local read "# of frames"() -> (w3901:i32)
                                n1238 = local read "refreshtime"() -> (w3893:dbl)
                                n1239 = local read "Pel"() -> (w3872:dbl)
                                n1240 = local read "bin"() -> (w3899:dbl)
                                n1241 = local read "Override AI buffer"() -> (w3870:bool)
                                n1242 = local read "finite samples"() -> (w3908:bool)
                                n1243 = local read "srateAODOtt"() -> (w3895:dbl)
                                n1244 = local read "srateAODOtt"() -> (w3902:dbl)
                                n1245 = local read "continuous"() -> (w3907:bool)
                                n1246 = local read "Angle ref"() -> (w3880:dbl)
                                n1247 = local read "wavdet"() -> (w3909:bool)
                                n1248 = local read "Vx-ref"() -> (w3904:dbl)
                                n1249 = local read "Vy-ref"() -> (w3906:dbl)
                                n1250 = local read "avpp"() -> (w3905:i32)
                                n1251 = call "tt_timeandsamples.vi"("bin"=w3899, "refreshtime"=w3893, "srateAODOtt"=w3896, "tot#ofsamples"=w3901) -> ("refreshrate"=w3897:dbl, "refreshbuffer"=w3898:i32, "timetracecycles"=w3903:i32)  [unwired: 5 in]
                                n1252 = local read "bin"() -> (w3900:dbl)
                                n1253 = call "2pparameters.vi"("command"="get") -> ("params out"=w3912:T10)  [unwired: 1 in]
                                n1254 = Bundle By Name(cluster=w3912, "Drawing Mode"=w3873, "measpoints"=w3901, "tt_cycles"=w3903, "refreshbuffer"=w3898, "refreshrate"=w3897, "Vx-ref"=w3904, "Vy-ref"=w3906, "srate"=w3895, "finite"=w3908, "cont"=w3907, "wavdet"=w3909, "avpp"=w3905, "srateAODO"=w3902, "bufferAI"=w3898, "bin"=w3900, "Angle Img"=w3880, "Vxminref"=w3879, "Vxmaxref"=w3878, "Vyminref"=w3877, "Vymaxref"=w3876, "Xpixels Img"=w3875, "Ypixels Img"=w3874, "Pel"=w3872, "Vz-reset"=0.0, "AIoverride"=w3870) -> (w3910:T10)
                                n1255 = Reciprocal(x=w3897) -> (1/x=w3894:dbl)
                                n1256 = local write "refreshtime"(w3894) -> ()
                                n1257 = call "2pparameters.vi"("Params in"=w3910, "command"="set") -> ()  [unwired: 1 out]
                                n1258 = local read "Voltage Clamp"() -> (w3887:bool)
                                n1259 = local read "Current Clamp"() -> (w3888:bool)
                                n1260 = local read "Vholding (mV)"() -> (w3882:sgl)
                                n1261 = local read "CC_ICgain"() -> (w3886:dbl)
                                n1262 = local read "OCgain"() -> (w3883:sgl)
                                n1263 = local read "holdon"() -> (w3881:bool)
                                n1264 = call "patchparameters.vi"("command"="get") -> ("Params out"=w3890:T13)  [unwired: 1 in]
                                n1265 = Bundle By Name(cluster=w3890, "VC"=w3887, "CC"=w3888, "CC_icg (pA/mv)"=w3886, "VC_icg (mV/mV)"=10.0, "OCG (mV/pA)"=w3883, "OVG (mV/mV)"=0.1, "Vhold (mV)"=w3882, "holdon"=w3881) -> (w3889:T13)
                                n1266 = call "patchparameters.vi"("Params in"=w3889, "command"="set") -> ()  [unwired: 1 out]
                              }
                              frame #4 {
                                n1267 = case shown="\"Point\"" w3914 {
                                frame "Point" {
                                n1268 = call "2pparameters.vi"("command"="get") -> ("params out"=w3930:T10)  [unwired: 1 in]
                                n1269 = Unbundle By Name(w3930) -> ("Pel"=w3919:sgl, "Vx-min Img"=w3932:dbl, "VX-max Img"=w3931:dbl, "Vy-min Img"=w3934:dbl, "Vy-max Img"=w3933:dbl, "Angle Img"=w3935:dbl, "Vx-ref"=w3928:dbl, "Vy-ref"=w3927:dbl)
                                n1270 = script code="Xic=(ximax+ximin)./2;\nYic=(yimax+yimin)./2;\nx=x-Xic;\ny=y-Yic;\nxout=x.*cos(pi/180.*phi)+y.*sin(pi./180.*phi)+Xic;\nyout=-x.*sin(pi./180.*phi)+y.*cos(pi./180.*phi)+Yic;"("ximax"=w3931, "ximin"=w3932, "yimax"=w3933, "yimin"=w3934, "phi"=w3935, "x"=w3928, "y"=w3927) -> ("xout"=w3921:dbl, "yout"=w3920:dbl)  [unwired: 1 in, 1 out]
                                n1271 = call "2pparameters.vi"("command"="get") -> ("params out"=w3923:T10)  [unwired: 1 in]
                                n1272 = Bundle By Name(cluster=w3923, "P"=0.0) -> (w3926:T10)
                                n1273 = Initialize Array(w3920, w3919) -> (w3917:dbl[])
                                n1274 = Initialize Array(w3921, w3919) -> (w3916:dbl[])
                                n1275 = call "2pparameters.vi"("Params in"=w3926, "command"="set") -> ()  [unwired: 1 out]
                                n1276 = call "X-array-databuffer.vi"("array in"=w3916, "command"=enum16{"get", "set", "clear", "append"}."set") -> ()  [unwired: 2 in, 2 out]
                                n1277 = call "Y-array-databuffer.vi"("array in"=w3917, "command"=enum16{"get", "set", "clear", "append"}."set") -> ()  [unwired: 2 in, 2 out]
                                }
                                frame "Resonant Ellipse", Default {
                                n1278 = call "2pparameters.vi"("command"="get") -> ("params out"=w3950:T10)  [unwired: 1 in]
                                n1279 = Unbundle By Name(w3950) -> ("srateAODO"=w3951:sgl, "Angle Img"=w3952:dbl, "Angle draw"=w3953:dbl, "Vxmaxref"=w3954:dbl, "Vxminref"=w3955:dbl, "Xpixels Img"=w3956:i32, "Ypixels Img"=w3957:i32, "Vymaxref"=w3958:dbl, "Vxminref"=w3959:dbl, "Drawing Mode"=w3960:u16, "Pel"=w3961:sgl)
                                n1280 = Add(x=w3952, y=w3953) -> (x+y=w3936:dbl)
                                n1281 = call "ROI-databuffer.vi"("command"=enum16{"get", "set", "clear", "append"}."get") -> ("array out"=w3944:cluster{"x":sgl, "y":sgl}[])  [unwired: 4 in]
                                n1282 = call "ScanningWaveform_v4.vi"("Vy-min"=w3959, "Vy-max"=w3958, "yPixels/tPixels"=w3957, "xPixels/rPixels"=w3956, "Vx-min"=w3955, "Vx-max"=w3954, "Drawing Mode"=w3960, "Angle"=w3936, "AOrate"=w3951, "Points"=w3944, "points in ellipse"=w3961) -> ("numPixels"=w3937:dbl, "Y-WaveArray"=w3938:dbl[], "P"=w3943:dbl, "X-WaveArray"=w3939:dbl[])  [unwired: 5 in]
                                n1283 = call "Y-array-databuffer.vi"("array in"=w3938, "command"=enum16{"get", "set", "clear", "append"}."set") -> ()  [unwired: 2 in, 2 out]
                                n1284 = call "X-array-databuffer.vi"("array in"=w3939, "command"=enum16{"get", "set", "clear", "append"}."set") -> ()  [unwired: 2 in, 2 out]
                                n1285 = call "2pparameters.vi"("command"="get") -> ("params out"=w3948:T10)  [unwired: 1 in]
                                n1286 = Bundle By Name(cluster=w3948, "P"=w3943, "sAOxy"=w3937, "Pel"=w3937) -> (w3940:T10)
                                n1287 = call "2pparameters.vi"("Params in"=w3940, "command"="set") -> ()  [unwired: 1 out]
                                }
                                }
                              }
                              frame #5 {
                                n1288 = call "X-array-databuffer.vi"("command"=enum16{"get", "set", "clear", "append"}."get") -> ("array out"=w3964:dbl[])  [unwired: 3 in, 1 out]
                                n1289 = call "Y-array-databuffer.vi"("command"=enum16{"get", "set", "clear", "append"}."get") -> ("array out"=w3967:dbl[])  [unwired: 3 in, 1 out]
                                n1290 = Index Array(array=w3964, index=0) -> (element=w3963:dbl)
                                n1291 = Index Array(array=w3967, index=0) -> (element=w3962:dbl)
                                n1292 = call "setposition.vi"("Vy"=w3962, "Vx"=w3963) -> ()  [unwired: 1 in]
                              }
                              frame #6 {
                                # "rem2Ps"
                                # "A2Ps"
                                # "Al"
                                # "Rl"
                                n1293 = stacked-sequence {
                                seq-local: [w3988 _ _ _ _ _ _ _ _ _ _] -> [_ w4100 _ w4161 _ w4247 _ _ _ _ _]
                                seq-local: [w3989 _ _ _ _ _ _ _ _ _ _] -> [_ w4101 w4111 _ w4216 _ _ _ _ _ _]
                                seq-local: [_ _ w4110 _ _ _ _ _ _ _ _] -> [_ _ _ _ w4210 _ _ _ _ _ _]
                                seq-local: [_ _ _ w4160 _ _ _ _ _ _ _] -> [_ _ _ _ _ w4246 _ _ _ _ _]
                                seq-local: [w3985 _ _ _ _ _ _ _ _ _ _] -> [_ w4097 _ _ _ _ _ _ w4432 w4500 _]
                                seq-local: [w3984 _ _ _ _ _ _ _ _ _ _] -> [_ w4096 _ _ _ _ _ _ w4433 w4501 _]
                                seq-local: [w3991 _ _ _ _ _ _ _ _ _ _] -> [_ _ _ _ _ _ w4285 _ w4431 w4499 _]
                                seq-local: [w3987 _ _ _ _ _ _ _ _ _ _] -> [_ w4095 _ _ _ _ w4284 w4352 _ _ _]
                                seq-local: [w3986 _ _ _ _ _ _ _ _ _ _] -> [_ w4094 _ _ _ _ w4283 w4351 _ _ _]
                                seq-local: [w3990 _ _ _ _ _ _ _ _ _ _] -> [_ _ _ _ _ _ w4282 w4350 _ _ _]
                                tunnel: [_ _ w4109 _ _ _ _ _ _ _ _] -> w3982
                                tunnel: [_ _ w4108 _ _ _ _ _ _ _ _] -> w3983
                                tunnel: [w3989 _ _ _ _ _ _ _ _ _ _] -> w3981
                                tunnel: [w3988 _ _ _ _ _ _ _ _ _ _] -> w3978
                                tunnel: [_ _ _ w4159 _ _ _ _ _ _ _] -> w3979
                                tunnel: [_ _ _ w4158 _ _ _ _ _ _ _] -> w3980
                                tunnel: [w3987 _ _ _ _ _ _ _ _ _ _] -> w3973
                                tunnel: [w3986 _ _ _ _ _ _ _ _ _ _] -> w3972
                                tunnel: [_ _ _ _ _ _ w4281 _ _ _ _] -> w3971
                                tunnel: [_ _ _ _ _ _ _ w4349 _ _ _] -> w3970
                                tunnel: [w3985 _ _ _ _ _ _ _ _ _ _] -> w3974
                                tunnel: [w3984 _ _ _ _ _ _ _ _ _ _] -> w3975
                                tunnel: [_ _ _ _ _ _ _ _ w4430 _ _] -> w3976
                                tunnel: [_ _ _ _ _ _ _ _ _ w4498 _] -> w3977
                                frame #0 {
                                # "for a next version, give ome thought to\nthe possibilit of intermittently updating the\nwaveforms. it will have to be a calculation\nbased on speed of CPU and program on the one hand\nand length of measurement on the other. but then it should be possible, in principle, to \nupdate the waveform on the fly and that way cut up a longer measurement in smaller parts."
                                n1294 = stacked-sequence {
                                tunnel: [w3992 _ _ _] -> w3989
                                tunnel: [_ w4004 _ _] -> w3988
                                tunnel: [_ _ _ w4061] -> w3984
                                tunnel: [_ _ _ w4060] -> w3985
                                tunnel: [_ _ _ w4059] -> w3991
                                tunnel: [_ _ w4019 _] -> w3987
                                tunnel: [_ _ w4018 _] -> w3986
                                tunnel: [_ _ w4017 _] -> w3990
                                frame #0 {
                                n1295 = call "configuration.vi"("command"="get") -> ("config out"=w3994:T11)  [unwired: 2 in, 1 out]
                                n1296 = Unbundle By Name(w3994) -> ("Voltage to Xgalvo"=w3993:i32)
                                n1297 = call "2pparameters.vi"("command"="get") -> ("params out"=w3998:T10)  [unwired: 1 in]
                                n1298 = in-place {
                                in-place-border: w3993 -> [w4003]
                                in-place-border: [w4000] -> w3992
                                n1299 = in-place-cluster #23(w3998) -> ("aAO"=w4002:u32[])
                                n1300 = call "add channel to active arrayv2.vi"("line array in"=w4002, "line to add"=w4003) -> ("line array out"=w4001:u32[], "addition"=w4000:bool)  [unwired: 1 out]
                                n1301 = in-place-cluster #23("aAO"=w4001) -> (w3996:T10)
                                }
                                n1302 = call "2pparameters.vi"("Params in"=w3996, "command"="set") -> ()  [unwired: 1 out]
                                }
                                frame #1 {
                                n1303 = call "configuration.vi"("command"="get") -> ("config out"=w4006:T11)  [unwired: 2 in, 1 out]
                                n1304 = Unbundle By Name(w4006) -> ("Voltage to Ygalvo"=w4005:i32)
                                n1305 = call "2pparameters.vi"("command"="get") -> ("params out"=w4010:T10)  [unwired: 1 in]
                                n1306 = in-place {
                                in-place-border: w4005 -> [w4015]
                                in-place-border: [w4012] -> w4004
                                n1307 = in-place-cluster #24(w4010) -> ("aAO"=w4014:u32[])
                                n1308 = call "add channel to active arrayv2.vi"("line array in"=w4014, "line to add"=w4015) -> ("line array out"=w4013:u32[], "addition"=w4012:bool)  [unwired: 1 out]
                                n1309 = in-place-cluster #24("aAO"=w4013) -> (w4008:T10)
                                }
                                n1310 = call "2pparameters.vi"("Params in"=w4008, "command"="set") -> ()  [unwired: 1 out]
                                }
                                frame #2 {
                                n1311 = call "2pparameters.vi"("command"="get") -> ("params out"=w4021:T10)  [unwired: 1 in]
                                n1312 = Unbundle By Name(w4021) -> ("autoshutter"=w4020:bool, "wavdet"=w4016:bool)
                                n1313 = case shown="False" w4020 {
                                tunnel: [w4026 w4046] -> w4019
                                tunnel: [w4025 FALSE ("removal")] -> w4018
                                tunnel: [w4024 w4044] -> w4017
                                tunnel: w4016 -> [w4023 _]
                                frame False {
                                n1314 = case shown="False" w4023 {
                                tunnel: [FALSE ("addition") FALSE ("addition")] -> w4026
                                tunnel: [w4028 FALSE ("removal")] -> w4025
                                tunnel: [w4027 _] -> w4024
                                frame False {
                                n1315 = call "configuration.vi"("command"="get") -> ("config out"=w4034:T11)  [unwired: 2 in, 1 out]
                                n1316 = Unbundle By Name(w4034) -> ("2P shutter"=w4031:i32)
                                n1317 = call "2pparameters.vi"("command"="get") -> ("params out"=w4032:T10)  [unwired: 1 in]
                                n1318 = in-place {
